vi "Append Page number HF.vi"(0 "PDF Report IN":T24(xcontrol), 2 "Header or footer":T1={"Start at page"=1, "H/F Alignment"=enum."LEFT - middle", "Page #"={"Text 1"="", "Text 2"="", "Text 3"=""}, "Font"={"Name"="", "Size"=12.0, "Color"=0, "Style"={"Bold"=FALSE, "Italic"=FALSE, "Underline"=FALSE, "Strikeout"=FALSE}}}, 11 "error in (no error)":errorcluster, 13 "Position":T7) -> (4 "PDF Report OUT":T24(xcontrol), 15 "error out":errorcluster)   [LabVIEW 2012]
doc: "Appends a <B>page number</B> in a column header (or footer). You can use this polymorphic VI to append a colomn to a header (or footer). The data type you wire to the <B>Header or footer</B> input determines the polymorphic instance to use.\n\nThe header (or footer) can be divided up into three columns. Each column has the same width. The number of header (or footer) that you add determines the number of columns.\n\n<B>FRANÇAIS</B>\nAjoute un <B>numéro de page</B> dans une colonne d'un en-tête (ou d'un pied de page). Vous pouvez utiliser ce VI polymorphique pour ajouter une colonne à un en-tête (ou un pied de page). Le type de variable que vous reliez au terminal <B>Header or footer</B> détermine l'instance polymorphique à utiliser.\n\nL'en-tête (ou le pied de page) peut être divisé en un maximum de trois colonnes. Chaque colonne a la même largeur. Le nombre d'en-têtes (ou de pieds de page) que vous ajoutez détermine le nombre de colonnes.\n\n\n\nVersion 1.0\nDeveloped by Jean-Marc Simard\nCopyright © 2010, Exaprom Inc.\nAll rights reserved.\nLicense: BSD\n\nWith iTextSharp 4.1.6 (http://itextsharp.sourceforge.net)\nunder Mozilla Public License Version 1.1\n(http://www.mozilla.org/MPL/MPL-1.1.html)"
uses:
  Controls/Header Footer Type.ctl
  Controls/Font color.ctl
  Controls/Header Footer Line.ctl
  Controls/Font size.ctl
  Controls/Font cluster.ctl
  Controls/Page number.ctl
  Controls/Cell Vertical alignment.ctl
  Controls/Header footer horiz alignment.ctl
  Controls/Header Footer cluster.ctl
  C:/Users/MaxCorp/Documents/GitHub/TopView/DLL/itextsharp.dll
  GitHub/TopView/DLL/itextsharp.dll
  Controls/H F Alignment.ctl
  Controls/Header or Footer.ctl
  Controls/PDF Report Xcontrol/PDF Report.xctl
  Controls/Header or Footer  Page # cluster.ctl
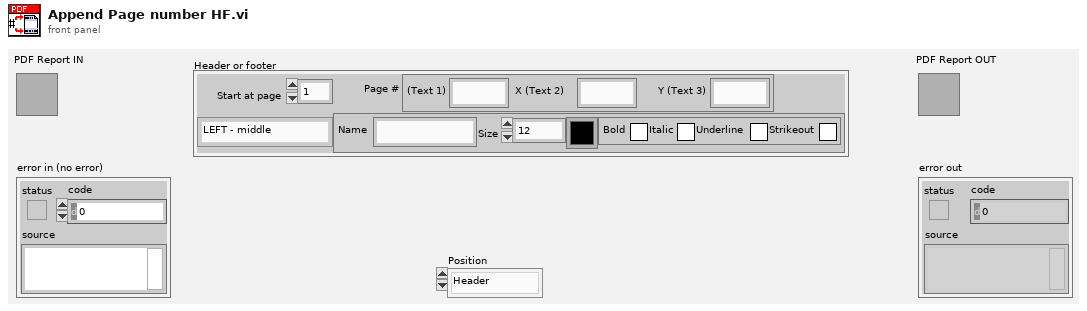
[diagram p1: front panel]
types:
  T1 = typedef "Header or Footer  Page # cluster.ctl" = cluster{"Start at page":i32, "H/F Alignment":T2, "Page #":T3, "Font":T4}
  T2 = typedef "H F Alignment.ctl" = enum16{"LEFT - top", "LEFT - middle", "LEFT - bottom", "CENTER - top", "CENTER - middle", "CENTER - bottom", "RIGHT - top", "RIGHT - middle", "RIGHT - bottom", ""}
  T3 = typedef "Page number.ctl" = cluster{"Text 1":string, "Text 2":string, "Text 3":string}
  T4 = typedef "Font cluster.ctl" = cluster{"Name":string, "Size":T5, "Color":T6, "Style":cluster{"Bold":bool, "Italic":bool, "Underline":bool, "Strikeout":bool}}
  T5 = typedef "Font size.ctl" = sgl
  T6 = typedef "Font color.ctl" = u32
  T7 = typedef "Header or Footer.ctl" = enum16{"Header", "Footer"}
  T8 = typedef "Unit.ctl" = enum16{"inch", "mm"}
  T9 = typedef "Paragraphe cluster.ctl" = cluster{" Aligment":T10, "Line spacing":T11}
  T10 = typedef "Texte alignement.ctl" = enum16{"Select", "CENTER", "JUSTIFY", "LEFT", "RIGHT"}
  T11 = typedef "Line spacing.ctl" = enum16{"Select", "1.0", "1.5", "2.0"}
  T12 = typedef "Page dimensions.ctl" = cluster{"Start at page":i32, "Orientation":T13, "widht":sgl, "height":sgl, "Margin left":sgl, "Margin right":sgl, "Margin top":sgl, "Margin bottom":sgl}
  T13 = typedef "Page Orientation.ctl" = enum16{"Portrait", "Landscape"}
  T14 = typedef "Image or Table Caption.ctl" = cluster{"Caption":string, "Separator":string, "Position":enum16{"Above", "Below"}}
  T15 = typedef "Header Footer [ ].ctl" = T16[]
  T16 = typedef "Header Footer cluster.ctl" = cluster{"Start page":i32, "Type":T17, "Alignment":T18, "Vertical Alignement":T19, "Image (%)":sgl, "Page #":T3, "Text":string, "Path":string, "Font":T4, "Font refnum":refnum<k24>, "Line":cluster{"Line":T20, "Thickness (points)":sgl, "Colour":T6}}
  T17 = typedef "Header Footer Type.ctl" = enum16{"Select", "Text", "Text + hyperlink", "Page number", "Image", "Image + hyperlink"}
  T18 = typedef "Header footer horiz alignment.ctl" = enum16{"Left", "Center", "Right"}
  T19 = typedef "Cell Vertical alignment.ctl" = enum16{"TOP", "MIDDLE", "BOTTOM"}
  T20 = typedef "Header Footer Line.ctl" = enum16{"No line", "Horizontal line"}
  T21 = typedef "Watermark cluster2.ctl" = cluster{"Show? (F)":bool, "Type":enum16{"Image", "Text"}, "Opacity (%)":sgl, "Rotate(°)":sgl, "Position":cluster{"Position":T22, "X":sgl, "Y":sgl}, "Image path":path, "Scaled(%)":sgl, "Image refnum":refnum<k24>, "Text":string, "Font":cluster{"Name":string, "Size":T5, "Color":T6}, "Font refnum":refnum<k24>, "Alignment":T18, "Automatic":bool}
  T22 = typedef "Watermark Position.ctl" = enum16{"Absolute", "Center (page)", "Center (text section)"}
  T23 = typedef "System Fonts.ctl" = cluster{"Font name [ ]":string[], "Font and file names [ ]":cluster{"Font name":string, "File name":string}[]}
  T24 = cluster{"Document":refnum<k24>, "Writer":refnum<k24>, "Default Font":refnum<k24>, "Default Font cluster":T4, "Path":path, "Unit (default = mm)":T8, "Paragraphe cluster":T9, "Pages dimensions [ ]":T12[], "Captions":cluster{"Image":T14, "Image counter":u16, "Table":T14, "Table counter":u16, "Font":T4}, "Header":T15, "Footer":T15, "Watermark ":T21, "Actual VI name":string, "System Fonts":T23}
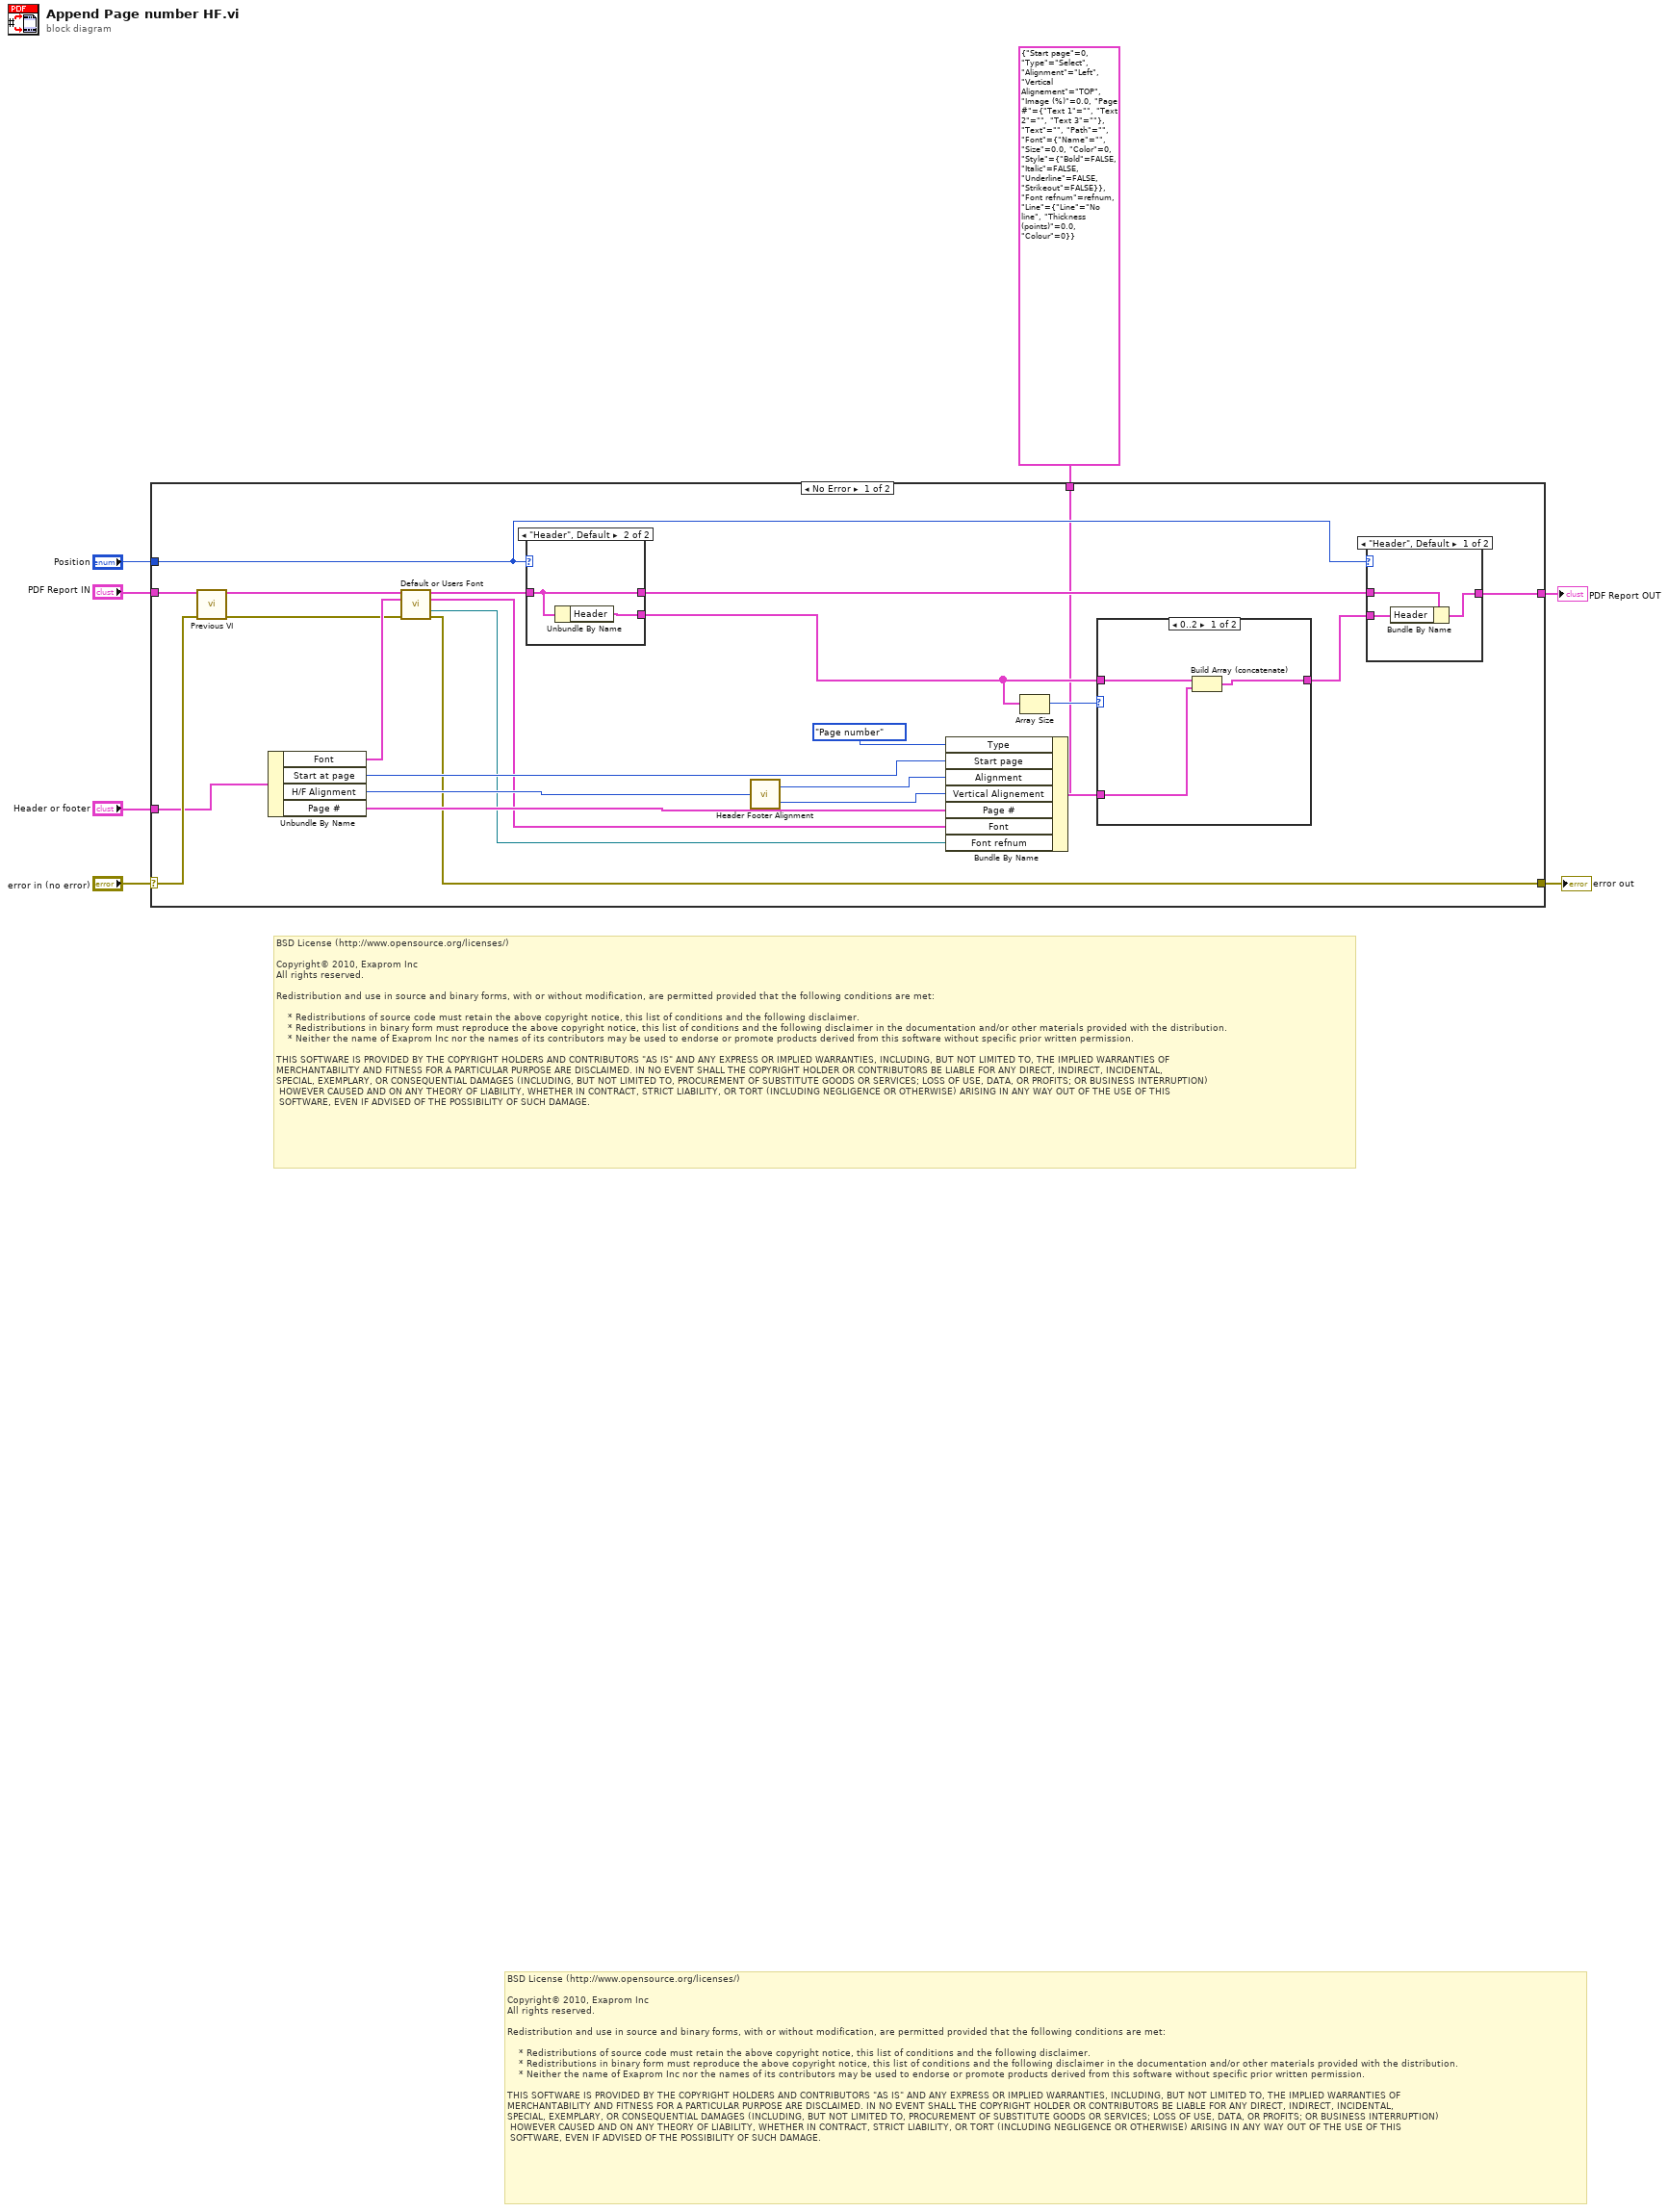
[diagram p0: block diagram]
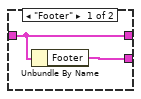
[diagram p3: hidden frame]
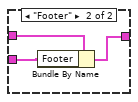
[diagram p4: hidden frame]
diagram:
  # "BSD License (http://www.opensource.org/licenses/)\n\nCopyright© 2010, Exaprom Inc\nAll rights reserved.\n\nRedistribution and use in source and binary forms, with or without modification, are permitted provided that the following conditions are met:\n\n    * Redistributions of source code must retain the above copyright notice, this list of conditions and the following disclaimer.\n    * Redistributions in binary form must reproduce the above copyright notice, this list of conditions and the following disclaimer in the documentation and/or other materials provided with the distribution.\n    * Neither the name of Exaprom Inc nor the names of its contributors may be used to endorse or promote products derived from this software without specific prior written permission.\n\nTHIS SOFTWARE IS PROVIDED BY THE COPYRIGHT HOLDERS AND CONTRIBUTORS \"AS IS\" AND ANY EXPRESS OR IMPLIED WARRANTIES, INCLUDING, BUT NOT LIMITED TO, THE IMPLIED WARRANTIES OF \nMERCHANTABILITY AND FITNESS FOR A PARTICULAR PURPOSE ARE DISCLAIMED. IN NO EVENT SHALL THE COPYRIGHT HOLDER OR CONTRIBUTORS BE LIABLE FOR ANY DIRECT, INDIRECT, INCIDENTAL,\nSPECIAL, EXEMPLARY, OR CONSEQUENTIAL DAMAGES (INCLUDING, BUT NOT LIMITED TO, PROCUREMENT OF SUBSTITUTE GOODS OR SERVICES; LOSS OF USE, DATA, OR PROFITS; OR BUSINESS INTERRUPTION)\n HOWEVER CAUSED AND ON ANY THEORY OF LIABILITY, WHETHER IN CONTRACT, STRICT LIABILITY, OR TORT (INCLUDING NEGLIGENCE OR OTHERWISE) ARISING IN ANY WAY OUT OF THE USE OF THIS\n SOFTWARE, EVEN IF ADVISED OF THE POSSIBILITY OF SUCH DAMAGE."
  # "BSD License (http://www.opensource.org/licenses/)\n\nCopyright© 2010, Exaprom Inc\nAll rights reserved.\n\nRedistribution and use in source and binary forms, with or without modification, are permitted provided that the following conditions are met:\n\n    * Redistributions of source code must retain the above copyright notice, this list of conditions and the following disclaimer.\n    * Redistributions in binary form must reproduce the above copyright notice, this list of conditions and the following disclaimer in the documentation and/or other materials provided with the distribution.\n    * Neither the name of Exaprom Inc nor the names of its contributors may be used to endorse or promote products derived from this software without specific prior written permission.\n\nTHIS SOFTWARE IS PROVIDED BY THE COPYRIGHT HOLDERS AND CONTRIBUTORS \"AS IS\" AND ANY EXPRESS OR IMPLIED WARRANTIES, INCLUDING, BUT NOT LIMITED TO, THE IMPLIED WARRANTIES OF \nMERCHANTABILITY AND FITNESS FOR A PARTICULAR PURPOSE ARE DISCLAIMED. IN NO EVENT SHALL THE COPYRIGHT HOLDER OR CONTRIBUTORS BE LIABLE FOR ANY DIRECT, INDIRECT, INCIDENTAL,\nSPECIAL, EXEMPLARY, OR CONSEQUENTIAL DAMAGES (INCLUDING, BUT NOT LIMITED TO, PROCUREMENT OF SUBSTITUTE GOODS OR SERVICES; LOSS OF USE, DATA, OR PROFITS; OR BUSINESS INTERRUPTION)\n HOWEVER CAUSED AND ON ANY THEORY OF LIABILITY, WHETHER IN CONTRACT, STRICT LIABILITY, OR TORT (INCLUDING NEGLIGENCE OR OTHERWISE) ARISING IN ANY WAY OUT OF THE USE OF THIS\n SOFTWARE, EVEN IF ADVISED OF THE POSSIBILITY OF SUCH DAMAGE."
  n1 = case shown="No Error" "error in (no error)" {
    selector: "error in (no error)" -> [w16 w47]
    tunnel: "PDF Report IN" -> [w17 w46]
    tunnel: "Position" -> [w28 _]
    tunnel: [w31 w46] -> w2
    tunnel: [w10 w47] -> w3
    tunnel: "Header or footer" -> [w15 _]
    tunnel: T16 {"Start page"=0, "Type"=enum."Select", "Alignment"=enum."Left", "Vertical Alignement"=enum."TOP", "Image (%)"=0.0, "Page #"={"Text 1"="", "Text 2"="", "Text 3"=""}, "Text"="", "Path"="", "Font"={"Name"="", "Size"=0.0, "Color"=0, "Style"={"Bold"=FALSE, "Italic"=FALSE, "Underline"=FALSE, "Strikeout"=FALSE}}, "Font refnum"=refnum, "Line"={"Line"=enum."No line", "Thickness (points)"=0.0, "Colour"=0}} ("element") -> [w18 _]
    frame No Error {
      n2 = call "Previous VI.vi"("PDF Report IN"=w17, "error in (no error)"=w16) -> ("PDF Report OUT"=w14:T24, "error out"=w11:errorcluster)  [unwired: 12 out]
      n3 = Unbundle By Name(w15) -> ("Font"=w12:T4, "Start at page"=w29:i32, "H/F Alignment"=w27:T2, "Page #"=w24:T3)
      n4 = call "Default or Users Font.vi"("PDF Report"=w14, "Font"=w12, "error in (no error)"=w11) -> ("PDF Report duplicate"=w13:T24, "Font OUT"=w9:T4, "Font Ref"=w8:refnum<k24>, "error out"=w10:errorcluster)  [unwired: 9 out]
      n5 = case shown="\"Header\", Default" w28 {
        tunnel: w13 -> [w37 w39]
        tunnel: [w37 w39] -> w30
        tunnel: [w36 w38] -> w19
        frame "Footer" {
          n6 = Unbundle By Name(w37) -> ("Footer"=w36:T15)
        }
        frame "Header", Default {
          n7 = Unbundle By Name(w39) -> ("Header"=w38:T15)
        }
      }
      n8 = call "Header Footer Alignment.vi"("H/F Alignment"=w27) -> ("Vertical Alignement"=w25:T19, "Horizontal Alignment"=w26:T18)  [unwired: 2 out]
      n9 = Bundle By Name(cluster=w18, "Type"=Header_Footer_Type."Page number", "Start page"=w29, "Alignment"=w26, "Vertical Alignement"=w25, "Page #"=w24, "Font"=w9, "Font refnum"=w8) -> (w21:T16)
      n10 = Array Size(array=w19) -> (size(s)=w20:i32)
      n11 = case shown="0..2" w20 {
        tunnel: w21 -> [w34 _]
        tunnel: [w32 w35] -> w22
        tunnel: w19 -> [w33 w35]
        frame 0..2 {
          n12 = Build Array (concatenate)(w33, w34) -> (w32:T15)
        }
        frame 3.., Default {
        }
      }
      n13 = case shown="\"Header\", Default" w28 {
        tunnel: w30 -> [w42 w45]
        tunnel: w22 -> [w40 w43]
        tunnel: [w41 w44] -> w31
        frame "Header", Default {
          n14 = Bundle By Name(cluster=w42, "Header"=w40) -> (w41:T24)
        }
        frame "Footer" {
          n15 = Bundle By Name(cluster=w45, "Footer"=w43) -> (w44:T24)
        }
      }
    }
    frame Error {
    }
  }
  "PDF Report OUT" <- w2
  "error out" <- w3
